vi "CSM MDI.vi"(7 "Name (\"\" to Use UUID)":string="Event CSM") -> ()   [LabVIEW 2020, in "MDI ViewManager.lvlib"]
uses:
  MDI ViewManager.lvlib
  Typedef/View.ctl
  <vilib>/Utility/miscctls.llb/LVPointTypeDef.ctl
  <vilib>/Utility/miscctls.llb/LVPoint32TypeDef.ctl
  Typedef/Update ViewList.ctl
  Typedef/LayoutMap.ctl
  <vilib>/Utility/miscctls.llb/LVBoundsTypeDef.ctl
  <vilib>/Utility/miscctls.llb/LVPositionTypeDef.ctl
  e08e3f9e-33cf-4499-bbf1-3a0f395d34a1.vi
  81b46446-0aca-48f9-86dc-ebdbbb8ef4b6.vi
  ccb737c0-95ef-485f-9e6a-728d6ff02605.vi
  5110686f-90b8-48a6-8112-abce107b1655.vi
  <userlib>/_NEVSTOP/Communicable State Machine(CSM)/AdvanceAPI/CSM - Revert Arguments-Safe String.vi
  <userlib>/_NEVSTOP/Communicable State Machine(CSM)/_Shared/Trim Single-line Text.vi
  <userlib>/_NEVSTOP/Communicable State Machine(CSM)/AdvanceAPI/CSM - Make String Arguments Safe.vi
  <userlib>/_NEVSTOP/Communicable State Machine(CSM)/AdvanceAPI/CSM - Break Down Multiple States String.vi
  <userlib>/_NEVSTOP/Communicable State Machine(CSM)/AdvanceAPI/CSM - Compact Multiple States.vi
  e08e3f9e-33cf-4499-bbf1-3a0f395d34a1.vi/b09b9099-6be0-413b-8afc-4908471460c3.vi
  <userlib>/_NEVSTOP/Communicable State Machine(CSM)/addons/INI-Static-Variable-Support/_Support/FlagInstance-CSMINIVariable.vi
  81b46446-0aca-48f9-86dc-ebdbbb8ef4b6.vi/99de0c97-112a-4c86-9094-c187659127e1.vi
  <userlib>/_NEVSTOP/Communicable State Machine(CSM)/AdvanceAPI/CSM - Keywords.vi
  <userlib>/_NEVSTOP/Communicable State Machine(CSM)/_Support/ChangeFlag/ChangeFlag-Read.vi
  <vilib>/Utility/cursorutil.llb/Set Cursor (Icon Pict).vi
  <userlib>/_NEVSTOP/Communicable State Machine(CSM)/_Support/ChangeFlag/ChangeFlagDB.vi
  <vilib>/Utility/Data Type/Get Type Information.vi
  <userlib>/_NEVSTOP/Communicable State Machine(CSM)/addons/API-String-Arugments-Support/_Support/Data To SingleElementsArray_csm.vi
  <userlib>/_NEVSTOP/Communicable State Machine(CSM)/addons/INI-Static-Variable-Support/_Support/Parse Used Session and Name.vi
  <userlib>/_NEVSTOP/Communicable State Machine(CSM)/addons/API-String-Arugments-Support/_Support/Data To API String Arguments.vi
  <userlib>/_NEVSTOP/Communicable State Machine(CSM)/addons/INI-Static-Variable-Support/_Support/INI-FGV(lvlibp).vi
  <userlib>/_NEVSTOP/Communicable State Machine(CSM)/addons/INI-Static-Variable-Support/_Support/Populate String with INI Variable.vi
  <userlib>/_NEVSTOP/Communicable State Machine(CSM)/addons/API-String-Arugments-Support/_Support/Convert API String Arguments to Data(variant).vi
  <userlib>/_NEVSTOP/Communicable State Machine(CSM)/addons/API-String-Arugments-Support/_Support/SingleElementsArray To Data_csm.vi
  <userlib>/_NEVSTOP/Communicable State Machine(CSM)/Communicable State Machine.lvlib
  <userlib>/_NEVSTOP/Communicable State Machine(CSM)/addons/INI-Static-Variable-Support/INI-Static-Variable-Support.lvlib
panel:
  in  "Tab Control 18":T1
  in  "Tab Control 17":T1
  in  "Tab Control 16":T1
  in  "Tab Control 15":T1
  in  "Tab Control 14":T1
  in  "Tab Control 13":T1
  in  "Tab Control 12":T1
  in  "Tab Control 11":T1
  in  "Tab Control 10":T1
  in  "Tab Control 9":T1
  in  "Tab Control 8":T1
  in  "Tab Control 7":T1
  in  "Tab Control 6":T1
  in  "Tab Control 5":T1
  in  "Tab Control 4":T1
  in  "Tab Control 3":T1
  in  "Tab Control 2":T1
  in  "Tab Control":T1
  out "State History":string
types:
  T1 = typedef "MDI ViewManager.lvlib/View.ctl" = enum32{"Page 1", "Page 2"}
  T2 = typedef "LVPointTypeDef.ctl" = cluster{"Horizontal":i16, "Vertical":i16}
  T3 = typedef "LVPoint32TypeDef.ctl" = cluster{"Horizontal":i32, "Vertical":i32}
  T4 = typedef "MDI ViewManager.lvlib/Update ViewList.ctl" = cluster{"Name":string, "VIPath":path, "Height(Default)":u32, "Widht(Default)":u32, "VIRef":refnum<vi>}
  T5 = typedef "MDI ViewManager.lvlib/LayoutMap.ctl" = cluster{"Origin":T2, "Layout":cluster{"Pane Dimension":T6, "Position":T7, "Label":string, "Visible":bool, "InsertedViewName":string}[]}
  T6 = typedef "LVBoundsTypeDef.ctl" = cluster{"Width":u32, "Height":u32}
  T7 = typedef "LVPositionTypeDef.ctl" = cluster{"Left":i32, "Top":i32}
  T8 = cluster{"Ref":cluster{"TabCtls":refnum<vi>[], "CurrMoveCtl":refnum<vi>, "Pane":refnum<vi>, "SubPanel":refnum<vi>, "Owning VI":refnum<vi>}, "Val":cluster{"TabCtlMove?":bool, "MouseOffset":T3, "ViewList":T4[], "map in":map{string, T5}}}
  T9 = cluster{"Current VI Reference":refnum<vi>, "Close Panel on Exit?":bool}
  T10 = cluster{"Core":cluster{"Current VI Reference":refnum<vi>, "Close Panel on Exit?":bool}, "1":cluster{"Ref":cluster{"TabCtls":refnum<vi>[], "CurrMoveCtl":refnum<vi>, "Pane":refnum<vi>, "SubPanel":refnum<vi>, "Owning VI":refnum<vi>}, "Val":cluster{"TabCtlMove?":bool, "MouseOffset":T3, "ViewList":T4[], "map in":map{string, T5}}}}
  T11 = enum32{"Invalid", "Standard", "Closed", "Hidden", "Minimized", "Maximized"}
  T12 = enum32{"invalid app kind", "Development System", "Run Time System", "Student Edition", "Embedded LabVIEW", "Evaluation", "Custom"}
  T13 = cluster{"TabCtl":refnum<vi>[], "Pane":refnum<vi>, "Variant":variant, "map in":map{string, T5}}
  T14 = cluster{"Pane":refnum<vi>, "ViewList":T4[], "TabCtls":refnum<vi>[], "map in":map{string, T5}}
  T15 = typedef "Communicable State Machine.lvlib/_CSM_Response Source Message.ctl" = cluster{"‘State":string, "’Arguments":string, "’Error":errorcluster}
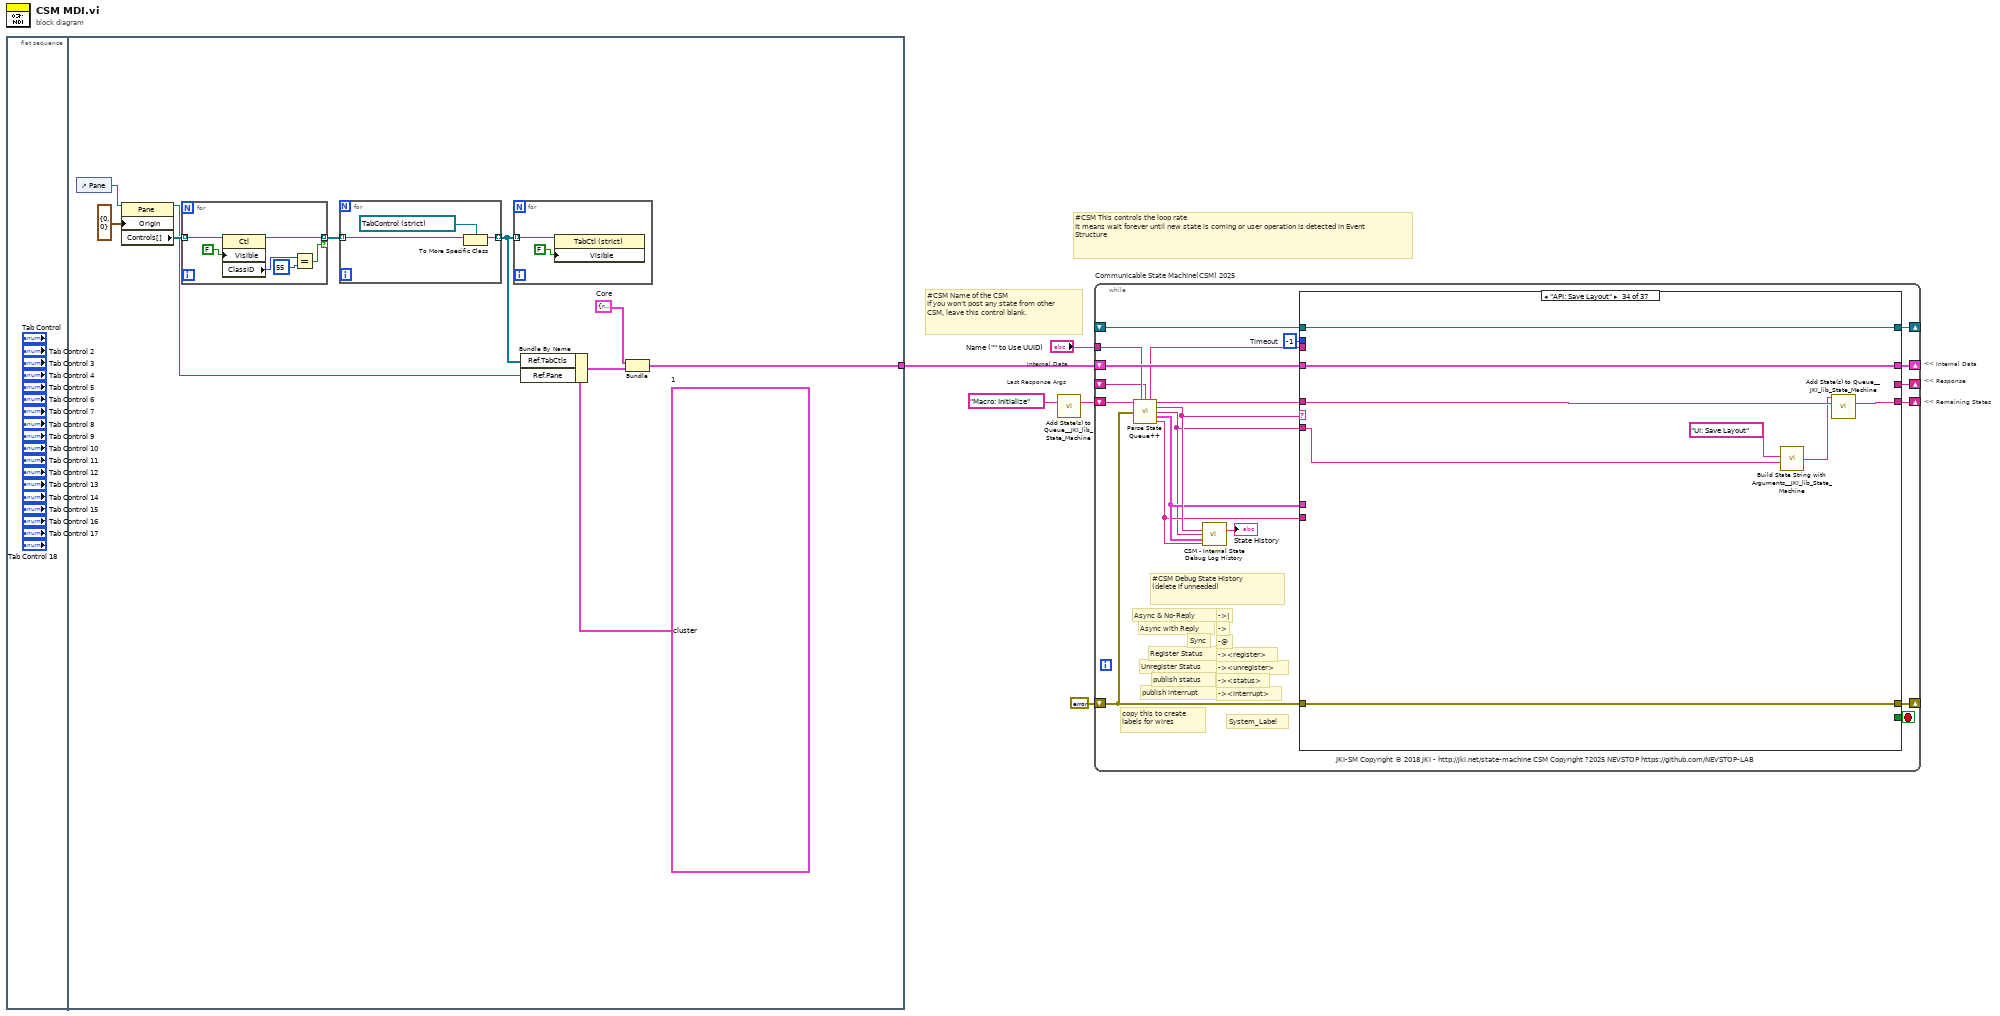
[diagram p0: block diagram]
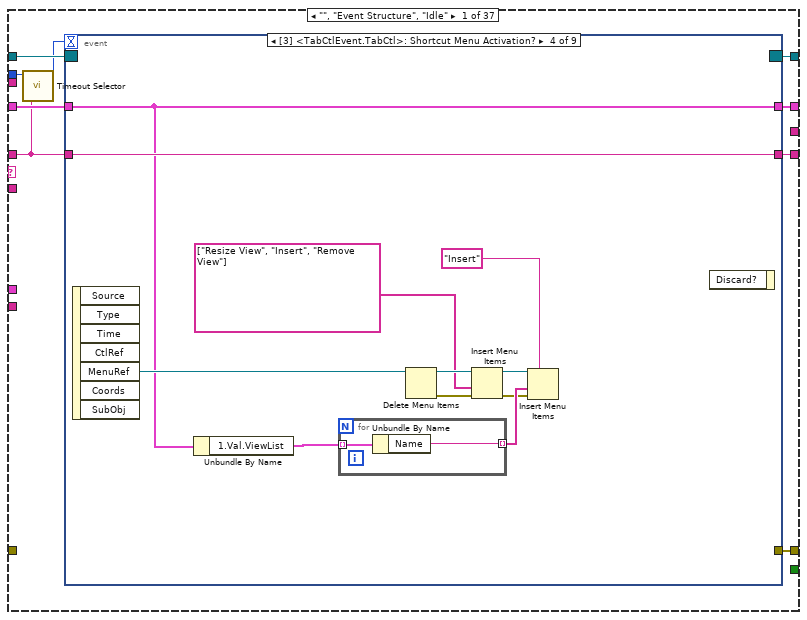
[diagram p2: hidden frame]
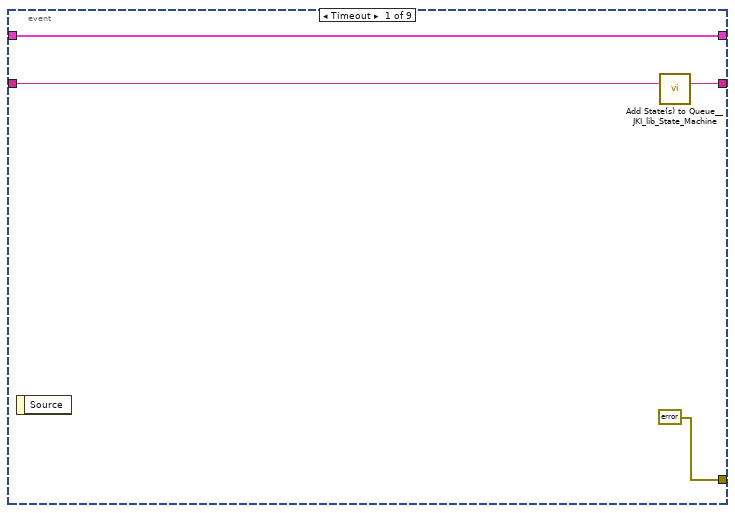
[diagram p3: hidden frame]
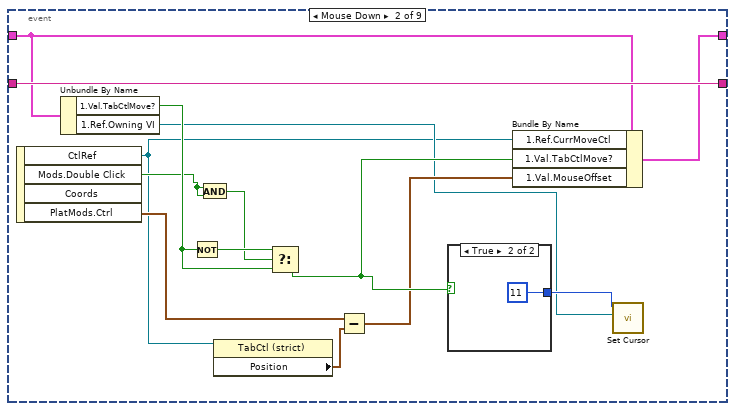
[diagram p4: hidden frame]
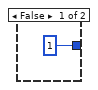
[diagram p5: hidden frame]
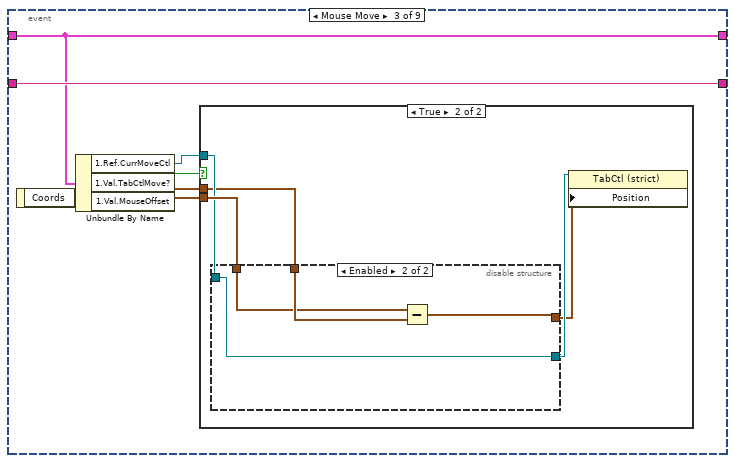
[diagram p6: hidden frame]
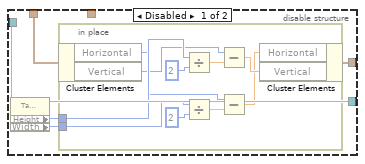
[diagram p8: hidden frame]
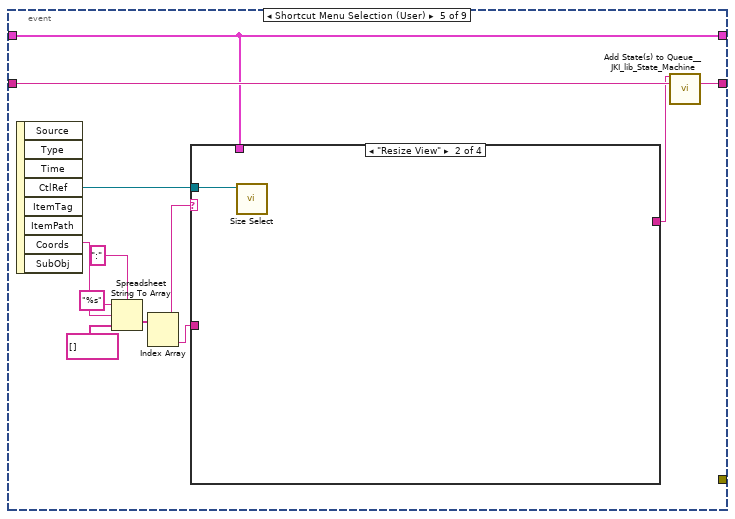
[diagram p9: hidden frame]
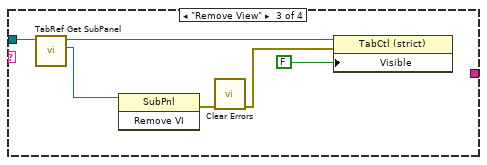
[diagram p11: hidden frame]
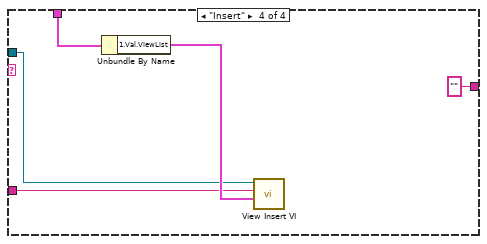
[diagram p12: hidden frame]
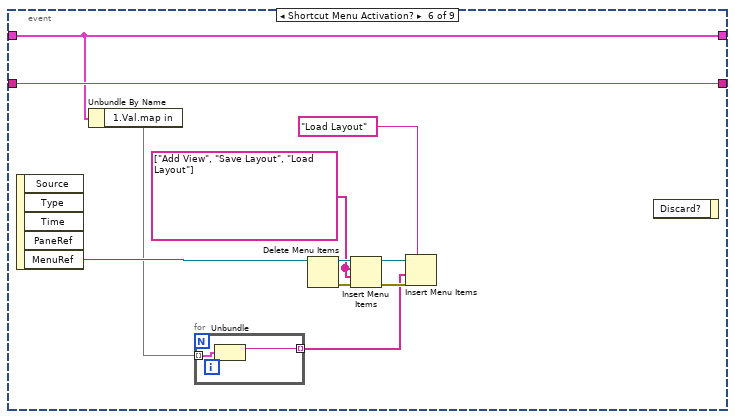
[diagram p13: hidden frame]
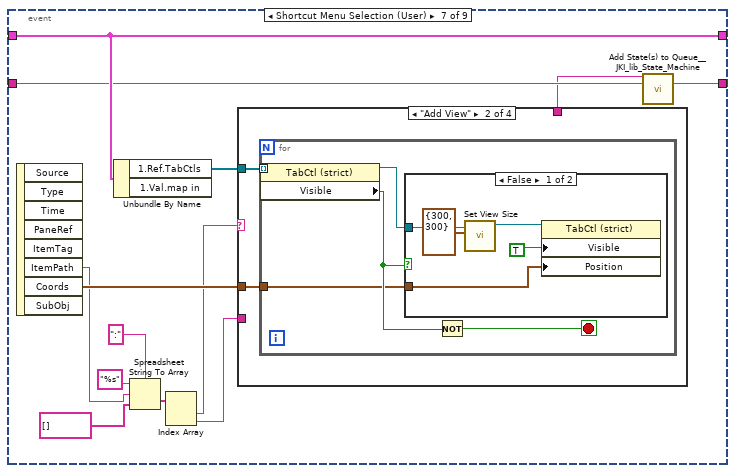
[diagram p14: hidden frame]
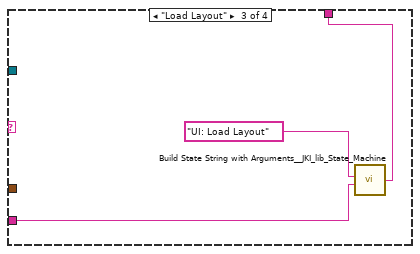
[diagram p17: hidden frame]
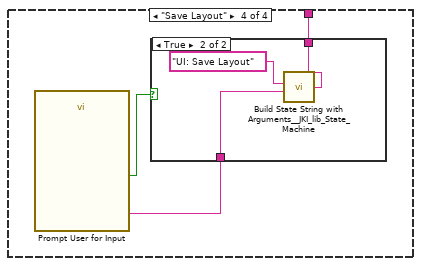
[diagram p18: hidden frame]
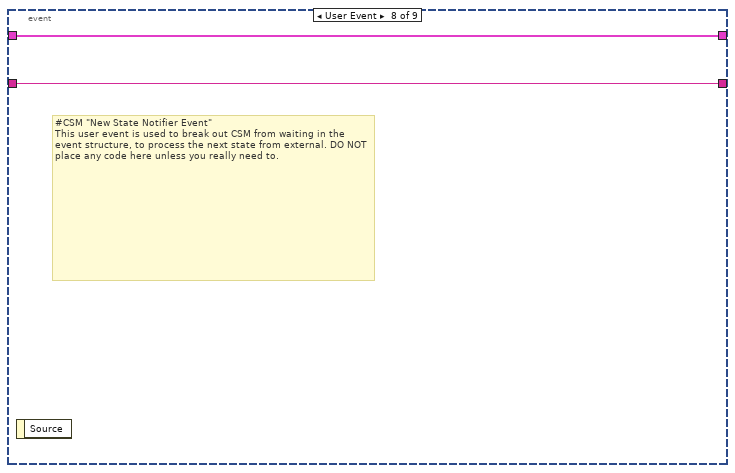
[diagram p20: hidden frame]
diagram:
  # "Last Response Args"
  # "Internal Data"
  # "<< Internal Data"
  # "<< Response"
  # "<< Remaining States"
  # "#CSM Name of the CSM\nIf you won't post any state from other CSM, leave this control blank."
  # "#CSM This controls the loop rate\nIt means wait forever until new state is coming or user operation is detected in Event Structure"
  n1 = flat-sequence {
    tunnel: [w15] -> w1
    frame #0 {
    }
    frame #1 {
      w13 = T8 {"Ref"={"TabCtls"=[], "CurrMoveCtl"=refnum, "Pane"=refnum, "SubPanel"=refnum, "Owning VI"=refnum}, "Val"={"TabCtlMove?"=FALSE, "MouseOffset"={"Horizontal"=0, "Vertical"=0}, "ViewList"=[], "map in"={}}}  # 1
      w12 = T9 {"Current VI Reference"=refnum, "Close Panel on Exit?"=FALSE}  # Core
      n2 = control-ref of="Pane"() -> (w9:refnum<vi>)
      n3 = property class="Pane"(reference=w9, "Origin"=T2 {"Horizontal"=0, "Vertical"=0}) -> (reference out=w6:refnum<vi>, "Controls[]"=w10:refnum<vi>[])  [unwired: 1 in, 1 out]
      n4 = for {
        tunnel: w10 -> [w24] mode=indexing
        tunnel: [w19] -> w8 mode=indexing if=w20
        n5 = property class="Ctl"(reference=w24, "Visible"=FALSE) -> (reference out=w19:refnum<vi>, "ClassID"=w22:u32)  [unwired: 1 in, 1 out]
        n6 = Equal?(x=w22, y=u32 55) -> (x = y?=w20:bool)
      }
      n7 = for {
        tunnel: w8 -> [w18] mode=indexing
        tunnel: [w17] -> w7 mode=indexing
        n8 = To More Specific Class(target class=refnum<vi> refnum ("Tab Control"), reference=w18) -> (specific class reference=w17:refnum<vi>)  [unwired: 1 in, 1 out]
      }
      n9 = for {
        tunnel: w7 -> [w25] mode=indexing
        n10 = property class="TabCtl (strict)"(reference=w25, "Visible"=FALSE) -> ()  [unwired: 1 in, 2 out]
      }
      n11 = Bundle By Name(cluster=w13, "Ref.TabCtls"=w7, "Ref.Pane"=w6) -> (w14:T8)
      n12 = Bundle("Core"=w12, "1"=w14) -> (w15:T10)  [unwired: 1 in]
    }
  }
  n13 = call <vilib>:"Add State(s) to Queue__JKI_lib_State_Machine.vi"("State(s) in (\"\")"="Macro: Initialize" ("Init State(\"Macro: Initialize\")")) -> ("States Out"=w2:string)  [unwired: 14 in]
  n14 = while "Communicable State Machine(CSM) 2025" {
    shift-right: [w41] -> _
    shift-left: w1 -> [w40]
    shift-right: [w44] -> _
    shift-left: errorcluster {"status"=FALSE, "code"=0, "source"=""} ("error out") -> [w38]
    shift-right: [w43] -> _
    shift-left: w2 -> [w45]
    tunnel: "Name (\"\" to Use UUID)" -> [w34]
    shift-right: [w37] -> _
    shift-left: _ -> [w29]
    shift-right: [w36] -> _
    shift-left: _ -> [w35]
    stop <- w42 stop-if-true
    w39 = -1  # Timeout
    # "#CSM Debug State History\n(delete if unneeded)"
    # "-><interrupt>"
    # "-><status>"
    # "-><unregister>"
    # "-><register>"
    # "-@"
    # "->"
    # "->|"
    # "publish interrupt"
    # "publish status"
    # "Unregister Status"
    # "Register Status"
    # "Sync"
    # "Async with Reply"
    # "Async & No-Reply"
    # "copy this to create labels for wires"
    # "System_Label"
    # "JKI-SM Copyright © 2018 JKI - http://jki.net/state-machine CSM Copyright ?2025 NEVSTOP https://github.com/NEVSTOP-LAB"
    n15 = call <userlib>:"Parse State Queue++.vi"("State Queue"=w45, "Name (\"\" to Use UUID)"=w34, "Response Arguments"=w29, "Previous Error"=w38) -> ("Name Used"=w30:string, "Remaining States"=w46:string, "Current State"=w33:string, "Arguments"=w28:string, "Additional Information"=w32:T15, "Source CSM"=w31:string)  [unwired: 6 in]
    n16 = call <userlib>:"CSM - Internal State Debug Log History.vi"("State"=w33, "Arguments (\"\")"=w28, ">> Response Source Message >>"=w32, "Source (\"\")"=w31) -> ("Debug Log"=→"State History":string)  [unwired: 11 in]
    n17 = case shown="\"API: Save Layout\"" w33 {
      selector: w33 -> [_ _ _ w214 _ _ _ _ _ _ _ _ _ _ _ _ _ _ _ _ _ _ _ _ _ _ _ _ _ _ _ _ _ _ _ _ _]
      tunnel: w46 -> [w48 w206 w211 w220 w226 w232 w258 w266 w273 w283 w292 w305 w310 w314 w322 w336 w340 w350 w354 w358 w362 w375 w387 w393 w404 w468 w473 w484 w487 w494 w499 w511 w514 w522 w531 w535 w539]
      tunnel: w28 -> [_ _ _ _ _ w230 w254 w261 w269 w277 _ _ _ _ _ _ _ _ _ _ _ w371 w378 w389 w399 _ _ _ _ w491 w496 w509 w515 w523 _ _ _]
      tunnel: w40 -> [w54 w205 w208 w218 w225 w238 w259 w264 w271 w281 w291 w299 w308 w312 w319 w332 w338 w342 w353 w356 w359 w370 w385 w391 w401 w466 w471 w482 w486 w493 w498 w505 w519 w527 w529 w533 w537]
      tunnel: [w53 _ w209 w212 w227 errorcluster {"status"=FALSE, "code"=0, "source"=""} ("error out") w251 w260 w267 w280 _ _ _ _ _ w333 _ w345 w352 _ _ w372 w376 w390 w402 _ _ _ _ _ _ _ w516 w524 _ _ _] -> w44
      tunnel: w38 -> [_ _ w209 w213 w227 w236 w252 w262 w268 _ _ _ _ _ _ w330 _ _ _ _ _ w373 w377 _ _ _ _ _ _ _ _ _ w516 w524 _ _ _]
      tunnel: [w55 w206 w210 w219 w226 w234 w257 w265 w272 w284 w292 w304 w309 w313 w321 w335 w339 w350 w354 w357 w361 w375 w387 w392 w403 w467 w472 w483 w487 w494 w499 w511 w513 w521 w530 w534 w538] -> w43
      tunnel: [_ _ _ _ _ _ TRUE _ _ _ _ _ TRUE _ _ _ _ _ _ _ _ _ _ _ _ _ _ _ _ _ _ _ _ _ _ _ _] -> w42
      tunnel: [w52 w205 w208 w218 w225 w238 w259 w264 w271 w282 w291 w303 w308 w312 w316 w332 w338 w342 w353 w356 w359 w364 w385 w391 w401 w466 w471 w482 w486 w489 w498 w503 w519 w527 w529 w533 w537] -> w41
      tunnel: w39 -> [w50 _ _ _ _ _ _ _ _ _ _ _ _ _ _ _ _ _ _ _ _ _ _ _ _ _ _ _ _ _ _ _ _ _ _ _ _]
      tunnel: w31 -> [_ _ _ _ _ w229 _ _ _ w278 _ _ _ _ _ _ _ _ _ _ _ _ _ _ _ _ _ _ _ _ _ _ _ _ _ _ _]
      tunnel: w32 -> [_ _ _ _ _ w228 _ _ _ w279 _ _ _ _ _ _ _ _ _ _ _ _ _ _ _ _ _ _ _ _ _ _ _ _ _ _ _]
      tunnel: [_ _ _ "" w221 _ _ _ _ _ _ _ _ _ _ _ _ _ _ _ _ _ _ _ _ _ _ _ _ _ _ _ _ _ _ _ _] -> w37
      tunnel: [w47 w204 w207 w216 w224 w237 w255 w263 w270 w285 w290 w293 w306 w311 w320 w331 w337 w349 w351 w355 w360 w374 w386 w388 w398 w465 w469 w475 w485 w492 w497 w510 w518 w526 w528 w532 w536] -> w36
      tunnel: w35 -> [w51 w204 w207 w216 w224 w237 w255 w263 w270 w285 w290 w293 w306 w311 w320 w331 w337 _ w351 w355 w360 w374 w386 w388 w398 w465 w469 w475 w485 w492 w497 w510 w518 w526 w528 w532 w536]
      tunnel: w30 -> [_ _ _ w215 _ _ w253 _ _ _ _ _ _ _ w317 w326 _ w348 _ _ _ _ _ _ _ _ _ _ _ _ _ _ _ _ _ _ _]
      frame "", "Event Structure", "Idle" {
        n18 = call <userlib>:"Timeout Selector.vi"("Remaining States"=w48, "Timeout Expected"=w50) -> ("Timeout"=w49:i32)  [unwired: 5 in]
        n19 = event shown="[3] <TabCtlEvent.TabCtl>: Shortcut Menu Activation?" {
          selector: w51 -> [_ _ _ _ _ _ _ _ _]
          dyn-events: [_ _ _ _ _ _ _ _ _] -> w47
          timeout: w49 -> [_ _ _ _ _ _ _ _ _]
          tunnel: w48 -> [w59 w73 w81 w117 w130 w154 w167 w191 w203]
          tunnel: [w58 w73 w81 w117 w129 w154 w166 w191 w202] -> w55
          tunnel: w54 -> [w57 w70 w79 w111 w120 w149 w169 w192 w201]
          tunnel: [errorcluster {"status"=FALSE, "code"=0, "source"=""} ("error out") _ _ _ _ _ _ _ _] -> w53
          tunnel: [w57 w68 w79 w111 w120 w149 w169 w192 w201] -> w52
          event Timeout {
            n20 = event-data() -> ()  [unwired: 1 in, 1 out]
            n21 = call <vilib>:"Add State(s) to Queue__JKI_lib_State_Machine.vi"("State(s) in (\"\")"=w59) -> ("States Out"=w58:string)  [unwired: 14 in]
          }
          event Mouse Down {
            n22 = event-data() -> ("CtlRef"=w60:refnum<vi>, "Mods.Double Click"=w61:bool, "Coords"=w65:T3)  [unwired: 1 in, 1 out]
            n23 = Unbundle By Name(w70) -> ("1.Val.TabCtlMove?"=w69:bool, "1.Ref.Owning VI"=w63:refnum<vi>)
            n24 = Not(x=w69) -> (.not. x?=w72:bool)
            n25 = And(x=w61, y=w61) -> (x .and. y?=w62:bool)
            n26 = property class="TabCtl (strict)"(reference=w60) -> ("Position"=w66:T7)  [unwired: 1 in, 2 out]
            n27 = Select(t=w72, s=w62, f=w69) -> (s? t:f=w67:bool)
            n28 = Subtract(x=w65, y=w66) -> (x-y=w64:T3)
            n29 = case shown="True" w67 {
              tunnel: [u16 1 ("icon") u16 11 ("icon")] -> w71
              frame False {
              }
              frame True {
              }
            }
            n30 = Bundle By Name(cluster=w70, "1.Ref.CurrMoveCtl"=w60, "1.Val.TabCtlMove?"=w67, "1.Val.MouseOffset"=w64) -> (w68:T10)
            n31 = call-poly <vilib>:"Set Cursor.vi"("VI reference (current VI)"=w63, "icon"=w71) -> ()  [unwired: 8 in, 2 out]
          }
          event Mouse Move {
            n32 = event-data() -> ("Coords"=w80:T3)  [unwired: 1 in]
            n33 = Unbundle By Name(w79) -> ("1.Ref.CurrMoveCtl"=w77:refnum<vi>, "1.Val.TabCtlMove?"=w78:bool, "1.Val.MouseOffset"=w76:T3)
            n34 = case shown="True" w78 {
              tunnel: w80 -> [_ w86]
              tunnel: w77 -> [_ w85]
              tunnel: w76 -> [_ w82]
              frame False {
              }
              frame True {
                n35 = disable-structure shown="Enabled" {
                  disable-tunnel: w86 -> [w90 w104]
                  disable-tunnel: w85 -> [w89 w106]
                  disable-tunnel: [w88 w106] -> w84
                  disable-tunnel: [w87 w103] -> w83
                  disable-tunnel: w82 -> [_ w105]
                  frame Disabled {
                    n36 = property class="TabCtl (strict)"(reference=w89) -> (reference out=w88:refnum<vi>, "Height"=w92:u32, "Width"=w91:u32)  [unwired: 1 in, 1 out]
                    n37 = in-place {
                      in-place-border: w92 -> [w102]
                      in-place-border: w91 -> [w96]
                      n38 = in-place-cluster #1(w90) -> ("Horizontal"=w94:i32, "Vertical"=w93:i32)
                      n39 = Divide(x=w102, y=u32 2) -> (x/y=w100:dbl)
                      n40 = Divide(x=w96, y=u32 2) -> (x/y=w97:dbl)
                      n41 = Subtract(x=w93, y=w100) -> (x-y=w99:dbl)
                      n42 = Subtract(x=w94, y=w97) -> (x-y=w95:dbl)
                      n43 = in-place-cluster #1("Horizontal"=w95, "Vertical"=w99) -> (w87:T3)
                    }
                  }
                  frame Enabled {
                    n44 = Subtract(x=w104, y=w105) -> (x-y=w103:T3)
                  }
                }
                n45 = property class="TabCtl (strict)"(reference=w84, "Position"=w83) -> ()  [unwired: 1 in, 2 out]
              }
            }
          }
          event Shortcut Menu Activation? {
            n46 = event-data() -> ("MenuRef"=w113:refnum<k9>)  [unwired: 1 in, 6 out]
            n47 = Unbundle By Name(w111) -> ("1.Val.ViewList"=w110:T4[])
            n48 = for {
              tunnel: w110 -> [w119] mode=indexing
              tunnel: [w118] -> w109 mode=indexing
              n49 = Unbundle By Name(w119) -> ("Name"=w118:string)
            }
            n50 = Delete Menu Items(9:w113) -> (0:w116:errorcluster, 3:w115:refnum<k9>)  [unwired: 3 in]
            n51 = Insert Menu Items(6:w116, 7:string[] ["Resize View", "Insert", "Remove View"] ("item names"), 9:w115) -> (0:w107:errorcluster, 3:w108:refnum<k9>)  [unwired: 3 in, 1 out]
            n52 = Insert Menu Items(5:"Insert", 6:w107, 7:w109, 9:w108) -> ()  [unwired: 2 in, 3 out]
            n53 = event-data() -> ()  [unwired: 2 in, 1 out]
          }
          event Shortcut Menu Selection (User) {
            n54 = event-data() -> ("CtlRef"=w131:refnum<vi>, "ItemPath"=w126:string)  [unwired: 1 in, 6 out]
            n55 = Spreadsheet String To Array(delimiter (Tab)=":", format string="%s", spreadsheet string=w126, array type (2D Dbl)=string[] [] ("delimiter (Tab)")) -> (array=w123:string[])
            n56 = Index Array(array=w123) -> (element #1=w122:string, element #2=w121:string)  [unwired: 2 in]
            n57 = case shown="\"Resize View\"" w122 {
              tunnel: w131 -> [_ w132 w138 w140]
              tunnel: [_ _ _ "" ("State(s) in Front (\"\")")] -> w128
              tunnel: w121 -> [_ _ _ w141]
              tunnel: w120 -> [_ _ _ w143]
              frame "False", Default {
              }
              frame "Resize View" {
                n58 = call "Size Select.vi"("CtlRef"=w132) -> ()  [unwired: 11 in]
              }
              frame "Remove View" {
                n59 = call "TabRef Get SubPanel.vi"("TabControl in"=w138) -> ("Sub Panel"=w134:refnum<vi>, "TabControl out"=w137:refnum<vi>)  [unwired: 8 in, 1 out]
                n60 = invoke class="SubPnl" method="Remove VI"(reference=w134) -> (error out=w135:errorcluster)  [unwired: 2 in, 2 out]
                n61 = call <vilib>:"Clear Errors.vi"("error in (no error)"=w135) -> ("error out"=w133:errorcluster)  [unwired: 5 in, 1 out]
                n62 = property class="TabCtl (strict)"(reference=w137, error in=w133, "Visible"=FALSE) -> ()  [unwired: 2 out]
              }
              frame "Insert" {
                n63 = Unbundle By Name(w143) -> ("1.Val.ViewList"=w142:T4[])
                n64 = call "View Insert VI.vi"("UpdateInsertableVI"=w142, "Name"=w141, "TabControl in"=w140) -> ()  [unwired: 9 in]
              }
            }
            n65 = call <vilib>:"Add State(s) to Queue__JKI_lib_State_Machine.vi"("State(s) in Front (\"\")"=w128, "State(s) in (\"\")"=w130) -> ("States Out"=w129:string)  [unwired: 13 in]
          }
          event Shortcut Menu Activation? {
            w151 = string[] ["Add View", "Save Layout", "Load Layout"] ("item names")
            n66 = event-data() -> ("MenuRef"=w150:refnum<k9>)  [unwired: 1 in, 4 out]
            n67 = Unbundle By Name(w149) -> ("1.Val.map in"=w148:map{string, T5})
            n68 = for {
              tunnel: w148 -> [w156] mode=indexing
              tunnel: [w155] -> w145 mode=indexing
              n69 = Unbundle(w156) -> (w155:string)  [unwired: 1 out]
            }
            n70 = Delete Menu Items(9:w150) -> (0:w153:errorcluster, 3:w152:refnum<k9>)  [unwired: 3 in]
            n71 = Insert Menu Items(6:w153, 7:w151, 8:w151, 9:w152) -> (0:w147:errorcluster, 3:w146:refnum<k9>)  [unwired: 2 in, 1 out]
            n72 = Insert Menu Items(5:"Load Layout", 6:w147, 7:w145, 9:w146) -> ()  [unwired: 2 in, 3 out]
            n73 = event-data() -> ()  [unwired: 2 in, 1 out]
          }
          event Shortcut Menu Selection (User) {
            n74 = event-data() -> ("ItemPath"=w160:string, "Coords"=w164:T3)  [unwired: 1 in, 6 out]
            n75 = Unbundle By Name(w169) -> ("1.Ref.TabCtls"=w168:refnum<vi>[])  [unwired: 1 out]
            n76 = Spreadsheet String To Array(delimiter (Tab)=":", format string="%s", spreadsheet string=w160, array type (2D Dbl)=string[] [] ("delimiter (Tab)")) -> (array=w161:string[])
            n77 = Index Array(array=w161) -> (element #1=w158:string, element #2=w157:string)  [unwired: 2 in]
            n78 = case shown="\"Add View\"" w158 {
              tunnel: w168 -> [_ w171 _ _]
              tunnel: w164 -> [_ w170 _ _]
              tunnel: [_ _ w182 w187] -> w165
              tunnel: w157 -> [_ _ w183 _]
              frame "False", Default {
              }
              frame "Add View" {
                n79 = for {
                  tunnel: w171 -> [w176] mode=indexing
                  tunnel: w170 -> [w172]
                  stop <- w174 stop-if-true
                  n80 = property class="TabCtl (strict)"(reference=w176) -> (reference out=w173:refnum<vi>, "Visible"=w175:bool)  [unwired: 1 in, 1 out]
                  n81 = case shown="False" w175 {
                    tunnel: w173 -> [w179 _]
                    tunnel: w172 -> [w180 _]
                    frame False {
                      n82 = call "Set View Size.vi"("TabDimension"=T6 {"Width"=300, "Height"=300}, "TabControlRef in"=w179) -> ("TabControlRef out"=w178:refnum<vi>)  [unwired: 8 in, 1 out]
                      n83 = property class="TabCtl (strict)"(reference=w178, "Visible"=TRUE, "Position"=w180) -> ()  [unwired: 1 in, 2 out]
                    }
                    frame True {
                    }
                  }
                  n84 = Not(x=w175) -> (.not. x?=w174:bool)
                }
              }
              frame "Load Layout" {
                n85 = call <vilib>:"Build State String with Arguments__JKI_lib_State_Machine.vi"("Arguments (\"\")"=w183, "State"="UI: Load Layout" ("State(s) in Front (\"\")")) -> ("State with Arguments"=w182:string)  [unwired: 4 in]
              }
              frame "Save Layout" {
                n86 = call "Prompt User for Input"() -> ("name"=w186:string, "OK"=w185:bool)  [unwired: 17 in, 1 out]
                n87 = case shown="True" w185 {
                  tunnel: [_ w189] -> w187
                  tunnel: w186 -> [_ w188]
                  frame False {
                  }
                  frame True {
                    n88 = call <vilib>:"Build State String with Arguments__JKI_lib_State_Machine.vi"("Arguments (\"\")"=w188, "State"="UI: Save Layout" ("State(s) in Front (\"\")")) -> ("State with Arguments"=w189:string)  [unwired: 4 in]
                  }
                }
              }
            }
            n89 = call <vilib>:"Add State(s) to Queue__JKI_lib_State_Machine.vi"("State(s) in Front (\"\")"=w165, "State(s) in (\"\")"=w167) -> ("States Out"=w166:string)  [unwired: 13 in]
          }
          event User Event {
            # "#CSM \"New State Notifier Event\"\nThis user event is used to break out CSM from waiting in the event structure, to process the next state from external. DO NOT place any code here unless you really need to."
            n90 = event-data() -> ()  [unwired: 1 in, 1 out]
          }
          event Panel Close? {
            # "#CSM Discard Panel Close?\nDiscard the event because we'll close the front panel ourselves in Macro: Exit"
            n91 = event-data() -> ()  [unwired: 1 in, 1 out]
            n92 = Call Chain() -> (call chain=w194:string[])
            n93 = Array Size(array=w194) -> (size(s)=w199:i32)
            n94 = Greater Or Equal?(x=w199, y=2) -> (x >= y?=w197:bool)
            n95 = Select(t="", s=w197, f="Macro: Exit") -> (s? t:f=w193:string)
            n96 = call <vilib>:"Add State(s) to Queue__JKI_lib_State_Machine.vi"("State(s) in Front (\"\")"=w193, "State(s) in (\"\")"=w203) -> ("States Out"=w202:string)  [unwired: 13 in]
            n97 = event-data("Discard?"=TRUE) -> ()  [unwired: 1 in, 1 out]
          }
        }
      }
      frame "CSM Documentation" {
        # "#CSM State Syntax\n\n// Comment line, all text to the right of “//” will be ignored\n// Local Message Example\nDoSth: DoA >> Arguments\n\n// Sync Call Example\nAPI: xxxx >> Arguments -@ TargetModule\n\n// Async Call Example\nAPI: xxxx >> Arguments -> TargetModule\n\n// Async Call without Reply Example\nAPI: xxxx >> Arguments ->| TargetModule\n\n// Broadcast normal status:\nStatus >> StatusArguments  -><status>\n\n// Broadcast Interrupt status:\nInterrupt >> StatusArguments  -><interrupt>\n\n// Register Source Module's status to Handler Module\nStatus@Source Module >> Handler Module@Handler Module -><register>\n\n// Unegister Source Module's status\nStatus@Source Module >> Handler Module -><unregister>"
        # "#CSM README FIRST\n\nCommunicable State Machine(CSM) is a LabVIEW application framework that builds upon JKI State Machine(JKISM). It follows the pattern of JKISM and extends the keywords to describe message communication between modules, including concepts such as Sync-Message, Async-Message, Subscription/Unsubscription of status - essential elements for creating reusable code modules. For more information, please visit the CSM wiki: https://nevstop-lab.github.io/CSM-Wiki/\n\nFor instructions on JKI State Machine, visit: \n    http://jki.net/state-machine/\nFor information about CSM, visit: \n    https://github.com/NEVSTOP-LAB"
        # "#CSM \"Documentation\"\nCase for holding CSM Documenation"
      }
      frame "---------- Core ----------" {
        # "#CSM \"Category Seperator\"\nDo not put any code in this frame."
        n98 = call <vilib>:"Add State(s) to Queue__JKI_lib_State_Machine.vi"("State(s) in (\"\")"=w211) -> ("States Out"=w210:string)  [unwired: 14 in]
      }
      frame Default {
        # "#CSM \"Default\"\nthis is used to capture unhandled states and typos"
        n99 = call <userlib>:"CSM Unhandled State Error.vi"("error in (no error)"=w213, "Undefined State"=w214, "CSM Name"=w215) -> ("error out"=w212:errorcluster)  [unwired: 8 in]
        n100 = call <vilib>:"Add State(s) to Queue__JKI_lib_State_Machine.vi"("State(s) in (\"\")"=w220) -> ("States Out"=w219:string)  [unwired: 14 in]
      }
      frame "VI Reference" {
        n101 = Unbundle By Name(w225) -> ("Core"=w223:T9)
        n102 = Unbundle By Name(w223) -> ("Current VI Reference"=w222:refnum<vi>)
        n103 = call <userlib>:"CSM - Convert Data to HexStr.vi"("Variant"=w222) -> ("HEX String (0-9,A-F)"=w221:string)  [unwired: 8 in]
      }
      frame "Error Handler" {
        # "#CSM Disable this error dialog if you need"
        # "#CSM \"Error Handler\"\nYou can also output any states to clean-up after errors occur"
        # "Clear error"
        n104 = case shown="Error" w236 {
          selector: w236 -> [_ w245]
          tunnel: [w243 w247] -> w233
          tunnel: w232 -> [w243 w246]
          tunnel: [w242 w245] -> w231
          tunnel: w230 -> [w244 _]
          tunnel: w229 -> [_ _]
          tunnel: w228 -> [_ _]
          frame No Error {
            n105 = call <userlib>:"CSM - Convert Argument to Error.vi"("Argument"=w244) -> ("Error"=w242:errorcluster)  [unwired: 4 in]
            n106 = flat-sequence {
              frame #0 {
                # "#CSM External Error Handler Case\nUsually, it's because This CSM register others' \"Error Occurred\" status with \"Error Handler\". If other CSM have any error, the error will be passed here for central handling."
              }
            }
          }
          frame Error {
            # "#CSM Internal Error Handler Case \nIf any error Occurred, \"Error Occurred\" \nstatus update will be broadcasted to system.\nParameter is Error Cluster."
            n107 = call <userlib>:"CSM - Convert Error to Argument.vi"("Error"=w245) -> ("Argument"=w249:string)  [unwired: 4 in]
            n108 = call <vilib>:"Build State String with Arguments__JKI_lib_State_Machine.vi"("Arguments (\"\")"=w249, "State"="Error Occurred" ("Status with Arguments")) -> ("State with Arguments"=w248:string)  [unwired: 4 in]
            n109 = call <userlib>:"CSM - Broadcast Status Change.vi"("Status With Arguments"=w248, "State Queue"=w246) -> ("Remaining States"=w247:string)  [unwired: 13 in]
          }
        }
        n110 = disable-structure shown="Enabled" {
          disable-tunnel: w231 -> [w240 w241]
          frame Enabled {
            # "Unhandled Error -- Display it"
            n111 = call <vilib>:"General Error Handler.vi"("error in (no error)"=w240) -> ()  [unwired: 10 in, 5 out]
          }
          frame Disabled {
            n112 = call <vilib>:"Clear Errors.vi"("error in (no error)"=w241) -> ()  [unwired: 5 in, 2 out]
          }
        }
        n113 = call <vilib>:"Add State(s) to Queue__JKI_lib_State_Machine.vi"("State(s) in Front (\"\")"="// Post Error States", "State(s) in (\"\")"=w233) -> ("States Out"=w234:string)  [unwired: 13 in]
      }
      frame "Critical Error" {
        # "#CSM \"Critical Error\"\nWhen any un-recoverable error occurs, CSM goes into this case."
        # "#CSM Stop in Critical Error\nWhen Critical Error occurs, Stop the loop immediately. Do NOT change this unless you fully understand the impact."
        n114 = call <userlib>:"CSM Critical Error.vi"("error in (no error)"=w252, "Arugments (As Reason)"=w254, "CSM Name"=w253) -> ("error out"=w251:errorcluster)  [unwired: 8 in]
        n115 = call <vilib>:"Add State(s) to Queue__JKI_lib_State_Machine.vi"("State(s) in (\"\")"=w258) -> ("States Out"=w257:string)  [unwired: 14 in]
      }
      frame "Target Timeout Error" {
        # "#CSM \"Target Timeout Error\"\nWhen This CSM could not get the sync-call response in time, This CSM goes into this case."
        n116 = call <userlib>:"CSM Target Timeout Error.vi"("error in (no error)"=w262, "Arguments (As CSM Name)"=w261) -> ("error out"=w260:errorcluster)  [unwired: 9 in]
        n117 = call <vilib>:"Add State(s) to Queue__JKI_lib_State_Machine.vi"("State(s) in (\"\")"=w266) -> ("States Out"=w265:string)  [unwired: 14 in]
      }
      frame "Target Error" {
        # "#CSM \"Target Error\"\nWhen This CSM try to communicate with an un-existed CSM, This CSM goes into this case."
        n118 = call <userlib>:"CSM Target Error.vi"("error in (no error)"=w268, "Arguments (As CSM Name)"=w269) -> ("error out"=w267:errorcluster)  [unwired: 9 in]
        n119 = call <vilib>:"Add State(s) to Queue__JKI_lib_State_Machine.vi"("State(s) in (\"\")"=w273) -> ("States Out"=w272:string)  [unwired: 14 in]
      }
      frame "Async Response", "Response" {
        # "#CSM \"Async Response\"\nHandle Async-call Response (\"Async Response\" for ->)"
        # "#CSM \"Response\"\nHandle Sync-call Response (\"Response\" for -@)"
        n120 = Unbundle(w279) -> ("‘State"=w276:string, "’Arguments"=w275:string, "’Error"=w274:errorcluster)
        n121 = case shown="Default" w276 {
          tunnel: [w286] -> w284
          tunnel: w283 -> [w287]
          tunnel: [w289] -> w282
          tunnel: w281 -> [w289]
          tunnel: [w288] -> w280
          tunnel: w274 -> [w288]
          tunnel: w278 -> [_]
          tunnel: w277 -> [_]
          tunnel: w275 -> [_]
          frame Default {
            # "#CSM Response Comments\nAfter Message is executed, CSM goes to this state for receive the response.\n    For Async Message(->), \"Async Response\" is used. This CSM will goes to \"Async Message Posted\" immediately and receive the \"Async Response\" after the callee finishes the message.\n    For Sync Message(@),  This CSM will wait until the message is done and immediately goes to \"Response\""
            n122 = call <vilib>:"Add State(s) to Queue__JKI_lib_State_Machine.vi"("State(s) in (\"\")"=w287) -> ("States Out"=w286:string)  [unwired: 14 in]
          }
        }
      }
      frame "Async Message Posted" {
        # "#CSM \"Async Message Posted\"\nAfter Async Message is posted (-> or ->| ), CSM goes to this state for post-action.\nYou can use Argument - State to tell which Async Message is called."
      }
      frame "Initialize Core Data" {
        # "#CSM \"Initialize Core Data\"\nThis is used to determine panel behavior on exit"
        # "originally closed?"
        # "exe?"
        # "If panel starts closed or is an EXE, then close it when we exit"
        n123 = property class="VI"() -> ("FP.State"=w296:T11)  [unwired: 2 in, 2 out]
        n124 = property class="App"() -> ("App.Kind"=w302:T12)  [unwired: 2 in, 2 out]
        n125 = control-ref of="Current VI Reference"() -> (w297:refnum<vi>)
        n126 = Equal?(x=w296, y=T11."Closed" ("Front Panel Window:State")) -> (x = y?=w294:bool)
        n127 = Equal?(x=w302, y=T12."Run Time System" ("Application:Kind")) -> (x = y?=w300:bool)
        n128 = Or(x=w294, y=w300) -> (x .or. y?=w298:bool)
        n129 = Bundle By Name(cluster=w299, "Core.Current VI Reference"=w297, "Core.Close Panel on Exit?"=w298) -> (w303:T10)
        n130 = call <vilib>:"Add State(s) to Queue__JKI_lib_State_Machine.vi"("State(s) in (\"\")"=w305) -> ("States Out"=w304:string)  [unwired: 14 in]
      }
      frame "Exit" {
        # "#CSM \"Exit\"\nCase for exiting the loop. No errors that occur here will be handled."
        n131 = call <vilib>:"Add State(s) to Queue__JKI_lib_State_Machine.vi"("State(s) in (\"\")"=w310) -> ("States Out"=w309:string)  [unwired: 14 in]
      }
      frame "---------- Data ----------" {
        # "#CSM \"Category Seperator\"\nDo not put any code in this frame."
        n132 = call <vilib>:"Add State(s) to Queue__JKI_lib_State_Machine.vi"("State(s) in (\"\")"=w314) -> ("States Out"=w313:string)  [unwired: 14 in]
      }
      frame "Data: Initialize" {
        n133 = Unbundle By Name(w319) -> ("1.Val.map in"=w318:map{string, T5})
        n134 = call "CSM - Read Configuration Variable.vim"("Section Name (\"\" as Default)"=w317, "Configuration Prototype (Cluster Prefered)"=w318) -> ("Configuration"=w315:map{string, T5})  [unwired: 6 in, 1 out]
        n135 = Bundle By Name(cluster=w319, "1.Val.map in"=w315) -> (w316:T10)
        n136 = call <vilib>:"Add State(s) to Queue__JKI_lib_State_Machine.vi"("State(s) in (\"\")"=w322) -> ("States Out"=w321:string)  [unwired: 14 in]
      }
      frame "Data: Cleanup" {
        w325 = TRUE ("All Temp Variable to Default Ini(F)")
        # "#CSM \"Data: Cleanup\"\nCleanup any data and references, here.\n(this is called automatically, by the Macro: Exit)"
        n137 = Unbundle By Name(w332) -> ("Core.Current VI Reference"=w334:refnum<vi>, "1.Ref.TabCtls"=w329:refnum<vi>[], "1.Val.map in"=w327:map{string, T5})
        n138 = call "CSM - Write Configuration Variable.vim"("Section Name (\"\" as Default)"=w326, "Configuration"=w327) -> ("error out"=w324:errorcluster)  [unwired: 6 in, 1 out]
        n139 = call <userlib>:"CSM - Mark All Temp Variables as Permanent.vi"("error in (no error)"=w324) -> ("error out"=w323:errorcluster)  [unwired: 8 in]
        n140 = call "Clean Layout.vi"("error in (no error)"=w330, "TabCtls"=w329) -> ("error out"=w328:errorcluster)  [unwired: 9 in]
        n141 = call <userlib>:"CSM - Sync Configuration Variables to File.vi"("Write UnSupported Datatype?(F)"=w325, "All Temp Variable to Default Ini(F)"=w325, "error in (no error)"=w323) -> ()  [unwired: 6 in, 1 out]
        n142 = Close Reference(reference=w334, error in (no error)=w328) -> (error out=w333:errorcluster)
        n143 = call <vilib>:"Add State(s) to Queue__JKI_lib_State_Machine.vi"("State(s) in (\"\")"=w336) -> ("States Out"=w335:string)  [unwired: 14 in]
      }
      frame "---------- Events ----------" {
        # "#CSM \"Category Seperator\"\nDo not put any code in this frame."
        n144 = call <vilib>:"Add State(s) to Queue__JKI_lib_State_Machine.vi"("State(s) in (\"\")"=w340) -> ("States Out"=w339:string)  [unwired: 14 in]
      }
      frame "Events: Register" {
        w344 = cluster{"TabCtl":refnum<vi>[]} {"TabCtl"=[]}  # TabCtlEvent
        # "#CSM \"Events: Register\"\nRegister user event. New Message Event is registered to break CSM waiting in event structure by default."
        # "#CSM Register New Message Event\nRegister message event to break Waiting in Event structure."
        n145 = Unbundle By Name(w342) -> ("1.Ref.TabCtls"=w341:refnum<vi>[])
        n146 = Bundle By Name(cluster=w344, "TabCtl"=w341) -> (w343:cluster{"TabCtl":refnum<vi>[]})
        n147 = call <userlib>:"CSM - Get New State Notifier Event.vi"("Name (\"\" to Use UUID)"=w348) -> ("error out"=w346:errorcluster, "New State Notifier Event"=w347:refnum<user-event>)  [unwired: 9 in]
        n148 = register-events(error in=w346, w347, w343, w343, w343) -> (reference out=w349:refnum<event-registration>, error out=w345:errorcluster)  [unwired: 1 in]
      }
      frame "Events: Unregister" {
        # "#CSM \"Events: Unregister\"\nUnregister user event."
        n149 = Unregister For Events(event registration refnum=w351) -> (error out=w352:errorcluster)  [unwired: 1 in]
      }
      frame "---------- UI ----------" {
        # "#CSM \"Category Seperator\"\nDo not put any code in this frame."
        n150 = call <vilib>:"Add State(s) to Queue__JKI_lib_State_Machine.vi"("State(s) in (\"\")"=w358) -> ("States Out"=w357:string)  [unwired: 14 in]
      }
      frame "UI: Initialize" {
        # "#CSM \"UI: Initialize\"\nInitialize the User Interface, here.\n(this is called automatically, by the Macro: Init)"
        n151 = call <vilib>:"Add State(s) to Queue__JKI_lib_State_Machine.vi"("State(s) in (\"\")"=w362) -> ("States Out"=w361:string)  [unwired: 14 in]
      }
      frame "UI: Save Layout" {
        n152 = Unbundle By Name(w370) -> ("1.Ref.TabCtls"=w367:refnum<vi>[], "1.Ref.Pane"=w366:refnum<vi>, "1.Val.map in"=w365:map{string, T5})
        n153 = Bundle By Name(cluster=T13 {"TabCtl"=[], "Pane"=refnum, "Variant"=variant, "map in"={}} ("input cluster"), "TabCtl"=w367, "Pane"=w366, "map in"=w365) -> (w368:T13)
        n154 = call "Save Layout.vi"("error in (no error)"=w373, "key"=w371, "input cluster"=w368) -> ("error out"=w372:errorcluster, "map out"=w363:map{string, T5})  [unwired: 7 in]
        n155 = Bundle By Name(cluster=w370, "1.Val.map in"=w363) -> (w364:T10)
      }
      frame "UI: Load Layout" {
        n156 = Unbundle By Name(w385) -> ("1.Ref.Pane"=w381:refnum<vi>, "1.Val.ViewList"=w382:T4[], "1.Ref.TabCtls"=w380:refnum<vi>[], "1.Val.map in"=w379:map{string, T5})
        n157 = Bundle By Name(cluster=T14 {"Pane"=refnum, "ViewList"=[], "TabCtls"=[], "map in"={}} ("Cluster"), "Pane"=w381, "ViewList"=w382, "TabCtls"=w380, "map in"=w379) -> (w383:T14)
        n158 = call "Load Layout By Name.vi"("error in (no error)"=w377, "key"=w378, "Cluster"=w383) -> ("error out"=w376:errorcluster)  [unwired: 8 in]
      }
      frame "UI: Cursor Set" {
        # "Argument"
        # "#CSM \"UI: Cursor Set\"\nSet and Unset Cursor Busy.\n(Usage: \"UI: Cursor Set >> Busy|Idle\")"
        n159 = disable-structure shown="Default" {
          disable-tunnel: [w395 _] -> w390
          disable-tunnel: w389 -> [w394 _]
          frame condition #0 (active) {
            n160 = case shown="\"Idle\", Default" w394 {
              tunnel: [w396 w397] -> w395
              frame "Idle", Default {
                n161 = call <vilib>:"Unset Busy.vi"() -> ("error out"=w396:errorcluster)  [unwired: 11 in]
              }
              frame "Busy" {
                n162 = call <vilib>:"Set Busy.vi"() -> ("error out"=w397:errorcluster)  [unwired: 10 in, 1 out]
              }
            }
          }
          frame condition #1 {
          }
        }
        n163 = call <vilib>:"Add State(s) to Queue__JKI_lib_State_Machine.vi"("State(s) in (\"\")"=w393) -> ("States Out"=w392:string)  [unwired: 14 in]
      }
      frame "UI: Front Panel State" {
        # "Argument"
        # "#CSM \"UI: Front Panel State\"\nSet Front Panel Open or Closed\n(Usage: \"UI: Front Panel State >> Open|Close\")"
        n164 = Unbundle By Name(w401) -> ("Core.Current VI Reference"=w400:refnum<vi>)
        n165 = case shown="\"Close\", \"Closed\"" w399 {
          tunnel: [w411 w424 w435 w447 w459] -> w402
          tunnel: w400 -> [w410 w422 w434 w446 w458]
          frame "Open", "Standard", Default {
            w405 = T11."Standard" ("State")
            n166 = property class="VI"(reference=w410) -> (reference out=w408:refnum<vi>, error out=w409:errorcluster, "FP.State"=w407:T11)  [unwired: 1 in]
            n167 = Not Equal?(x=w407, y=w405) -> (x != y?=w406:bool)
            n168 = case shown="True" w406 {
              tunnel: [w415 w417] -> w411
              tunnel: w409 -> [w414 w417]
              tunnel: w408 -> [w413 _]
              tunnel: w405 -> [w412 _]
              frame True {
                n169 = invoke class="VI" method="FP.Open"(reference=w413, error in=w414, "Activate"=TRUE, "State"=w412) -> (error out=w415:errorcluster)  [unwired: 1 in, 4 out]
              }
              frame False {
              }
            }
          }
          frame "Close", "Closed" {
            n170 = property class="VI"(reference=w422) -> (reference out=w421:refnum<vi>, error out=w423:errorcluster, "FP.State"=w419:T11)  [unwired: 1 in]
            n171 = Not Equal?(x=w419, y=T11."Closed" ("Front Panel Window:State")) -> (x != y?=w418:bool)
            n172 = case shown="True" w418 {
              tunnel: [w425 w428] -> w424
              tunnel: w423 -> [w425 w427]
              tunnel: w421 -> [_ w426]
              frame False {
              }
              frame True {
                n173 = invoke class="VI" method="FP.Close"(reference=w426, error in=w427) -> (error out=w428:errorcluster)  [unwired: 1 in, 2 out]
              }
            }
          }
          frame "Hidden", "Hide" {
            w429 = T11."Hidden" ("State")
            n174 = property class="VI"(reference=w434) -> (reference out=w432:refnum<vi>, error out=w433:errorcluster, "FP.State"=w431:T11)  [unwired: 1 in]
            n175 = Not Equal?(x=w431, y=w429) -> (x != y?=w430:bool)
            n176 = case shown="True" w430 {
              tunnel: [w439 w440] -> w435
              tunnel: w433 -> [w438 w440]
              tunnel: w432 -> [w437 _]
              tunnel: w429 -> [w436 _]
              frame True {
                n177 = invoke class="VI" method="FP.Open"(reference=w437, error in=w438, "State"=w436) -> (error out=w439:errorcluster)  [unwired: 2 in, 4 out]
              }
              frame False {
              }
            }
          }
          frame "Minimize", "Minimized" {
            w441 = T11."Minimized" ("State")
            n178 = property class="VI"(reference=w446) -> (reference out=w444:refnum<vi>, error out=w445:errorcluster, "FP.State"=w443:T11)  [unwired: 1 in]
            n179 = Not Equal?(x=w443, y=w441) -> (x != y?=w442:bool)
            n180 = case shown="False" w442 {
              tunnel: [w451 w452] -> w447
              tunnel: w445 -> [w450 w452]
              tunnel: w444 -> [w449 _]
              tunnel: w441 -> [w448 _]
              frame True {
                n181 = invoke class="VI" method="FP.Open"(reference=w449, error in=w450, "State"=w448) -> (error out=w451:errorcluster)  [unwired: 2 in, 4 out]
              }
              frame False {
              }
            }
          }
          frame "Maximize", "Maximized" {
            w453 = T11."Maximized" ("State")
            n182 = property class="VI"(reference=w458) -> (reference out=w456:refnum<vi>, error out=w457:errorcluster, "FP.State"=w455:T11)  [unwired: 1 in]
            n183 = Not Equal?(x=w455, y=w453) -> (x != y?=w454:bool)
            n184 = case shown="True" w454 {
              tunnel: [w463 w464] -> w459
              tunnel: w457 -> [w462 w464]
              tunnel: w456 -> [w461 _]
              tunnel: w453 -> [w460 _]
              frame True {
                n185 = invoke class="VI" method="FP.Open"(reference=w461, error in=w462, "State"=w460) -> (error out=w463:errorcluster)  [unwired: 2 in, 4 out]
              }
              frame False {
              }
            }
          }
        }
        n186 = call <vilib>:"Add State(s) to Queue__JKI_lib_State_Machine.vi"("State(s) in (\"\")"=w404) -> ("States Out"=w403:string)  [unwired: 14 in]
      }
      frame "---------- Macro ----------" {
        # "#CSM \"Category Seperator\"\nDo not put any code in this frame."
        n187 = call <vilib>:"Add State(s) to Queue__JKI_lib_State_Machine.vi"("State(s) in (\"\")"=w468) -> ("States Out"=w467:string)  [unwired: 14 in]
      }
      frame "Macro: Initialize" {
        w470 = "Data: Initialize\nInitialize Core Data\nUI: Initialize\nUI: Front Panel State >> Maximize\nEvents: Register\n//UI: Front Panel State >> Open"  # Data: Initialize Initialize Core Data UI: Initialize UI: Front Panel State >> Maximize Events: Register //UI: Front Panel State >> Open
        # "#CSM \"Macro: Initialize\"\nInitialization Macro (This is called once, when the VI starts)"
        n188 = call <vilib>:"Add State(s) to Queue__JKI_lib_State_Machine.vi"("State(s) in Front (\"\")"=w470, "State(s) in (\"\")"=w473) -> ("States Out"=w472:string)  [unwired: 13 in]
      }
      frame "Macro: Exit" {
        # "#CSM \"Macro: Exit\"\nExit Macro (This is called once, when the VI exits)"
        n189 = Unbundle By Name(w482) -> ("Core.Close Panel on Exit?"=w481:bool)
        n190 = Select(t="UI: Front Panel State >> Close", s=w481, f="") -> (s? t:f=w478:string)
        n191 = call <vilib>:"Add State(s) to Queue__JKI_lib_State_Machine.vi"("State(s) in Front (\"\")"="//Exit Sub-Modules ", "State(s) in (\"\")"=w478, "State(s) at Back (\"\")"="Data: Cleanup\nEvents: Unregister\nExit") -> ("States Out"=w476:string)  [unwired: 12 in]
        n192 = call <vilib>:"Add State(s) to Queue__JKI_lib_State_Machine.vi"("State(s) in Front (\"\")"=w476, "State(s) in (\"\")"=w484) -> ("States Out"=w483:string)  [unwired: 13 in]
      }
      frame "---------- API ----------" {
        # "#CSM \"Category Seperator\"\nDo not put any code in this frame."
      }
      frame "API: Update ViewList" {
        # "#CSM API Example\nCopy/Rename this case for your own API"
        n193 = call "Convert API String Arguments to Data.vim"("Reference Type"=T4[] [], "API String"=w491) -> ("Data"=w488:T4[])  [unwired: 6 in, 1 out]
        n194 = Bundle By Name(cluster=w493, "1.Val.ViewList"=w488) -> (w489:T10)
      }
      frame "API: Hello" {
        # "#CSM API Example\nCopy/Rename this case for your own API"
        n195 = Empty String/Path?(string/path=w496) -> (empty?=w495:bool)
        n196 = case shown="False" w495 {
          tunnel: w496 -> [w500 _]
          frame False {
            n197 = One Button Dialog(message=w500) -> ()  [unwired: 1 in, 1 out]
          }
          frame True {
          }
        }
      }
      frame "API: Update Subpanel" {
        # "#CSM API Example\nCopy/Rename this case for your own API"
        n198 = control-ref of="Sub Panel"() -> (w508:refnum<vi>)
        n199 = Unbundle By Name(w505) -> ("Core.Current VI Reference"=w504:refnum<vi>)
        n200 = call "Convert API String Arguments to Data.vim"("Reference Type"=w508, "API String"=w509) -> ("Data"=w502:refnum<vi>)  [unwired: 6 in, 1 out]
        n201 = property class="SubPnl"(reference=w502) -> ("OwningVI"=w501:refnum<vi>)  [unwired: 1 in, 2 out]
        n202 = invoke on="Invoke Node" class="VI" method="FP.Close"(reference=w504) -> (reference out=w506:refnum<vi>, error out=w507:errorcluster)  [unwired: 2 in, 1 out]
        n203 = invoke on="Invoke Node" class="SubPnl" method="Insert VI"(reference=w502, error in=w507, "VI Ref"=w506) -> ()  [unwired: 1 in, 4 out]
        n204 = Bundle By Name(cluster=w505, "1.Ref.Owning VI"=w501) -> (w503:T10)
      }
      frame "API: Load Layout" {
        n205 = call <vilib>:"Build State String with Arguments__JKI_lib_State_Machine.vi"("Arguments (\"\")"=w515, "State"="UI: Load Layout") -> ("State with Arguments"=w512:string)  [unwired: 4 in]
        n206 = call <vilib>:"Add State(s) to Queue__JKI_lib_State_Machine.vi"("State(s) in Front (\"\")"=w512, "State(s) in (\"\")"=w514) -> ("States Out"=w513:string)  [unwired: 13 in]
      }
      frame "API: Save Layout" {
        n207 = call <vilib>:"Build State String with Arguments__JKI_lib_State_Machine.vi"("Arguments (\"\")"=w523, "State"="UI: Save Layout") -> ("State with Arguments"=w520:string)  [unwired: 4 in]
        n208 = call <vilib>:"Add State(s) to Queue__JKI_lib_State_Machine.vi"("State(s) in Front (\"\")"=w520, "State(s) in (\"\")"=w522) -> ("States Out"=w521:string)  [unwired: 13 in]
      }
      frame "---------- Action ----------" {
        # "#CSM \"Category Seperator\"\nDo not put any code in this frame."
        n209 = call <vilib>:"Add State(s) to Queue__JKI_lib_State_Machine.vi"("State(s) in (\"\")"=w531) -> ("States Out"=w530:string)  [unwired: 14 in]
      }
      frame "Action: action1" {
        # "#CSM \"Internal State\"\nThis category is used for holding internal states"
        n210 = call <vilib>:"Add State(s) to Queue__JKI_lib_State_Machine.vi"("State(s) in (\"\")"=w535) -> ("States Out"=w534:string)  [unwired: 14 in]
      }
      frame "Action: action2" {
        # "#CSM \"Internal State\"\nThis category is used for holding internal states"
        n211 = call <vilib>:"Add State(s) to Queue__JKI_lib_State_Machine.vi"("State(s) in (\"\")"=w539) -> ("States Out"=w538:string)  [unwired: 14 in]
      }
    }
  }
